vi "Test_Split.vi"() -> ()   [LabVIEW 2021]
panel:
  in  "OK Button":bool
  in  "milliseconds to wait":u32
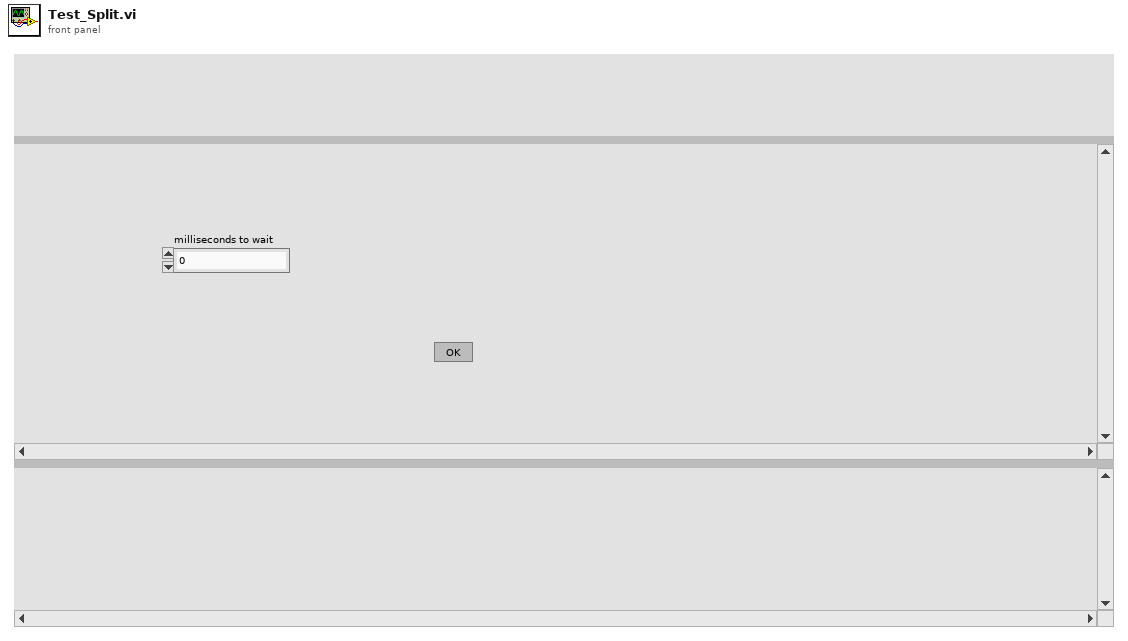
[diagram p1: front panel]
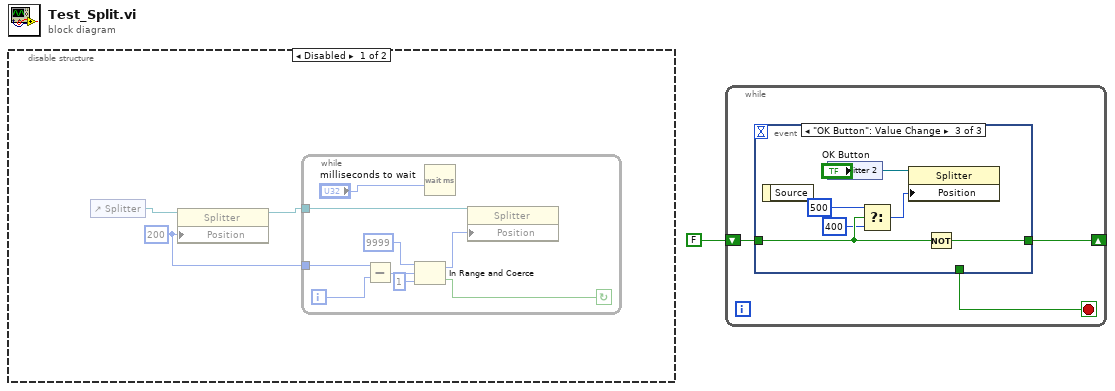
[diagram p0: block diagram]
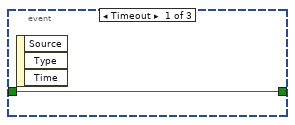
[diagram p2: hidden frame]
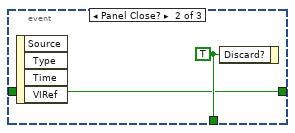
[diagram p3: hidden frame]
diagram:
  n1 = disable-structure shown="Disabled" {
    frame Disabled {
      w2 = 200 ("Splitter Position")
      n2 = control-ref of="Splitter"() -> (w4:refnum<vi>)
      n3 = property class="Splitter"(reference=w4, "Position"=w2) -> (reference out=w3:refnum<vi>)  [unwired: 1 in, 1 out]
      n4 = while {
        tunnel: w3 -> [w13]
        tunnel: w2 -> [w12]
        i -> [w11]
        stop <- w6 continue-if-true
        n5 = Subtract(x=w12, y=w11) -> (x-y=w10:i32)
        n6 = In Range and Coerce(upper limit=9999, x=w10, lower limit=1) -> (coerced(x)=w9:i32, In Range?=w6:bool)
        n7 = Wait (ms)(milliseconds to wait="milliseconds to wait") -> ()  [unwired: 1 out]
        n8 = property class="Splitter"(reference=w13, "Position"=w9) -> ()  [unwired: 1 in, 2 out]
      }
    }
    frame Enabled {
    }
  }
  n9 = while {
    shift-right: [w14] -> _
    shift-left: FALSE -> [w15]
    stop <- w16 stop-if-true
    n10 = event shown="[2] \"OK Button\": Value Change" {
      selector: _ -> [_ _ _]
      dyn-events: _ -> [_ _ _]
      timeout: _ -> [_ _ _]
      tunnel: [_ w19 _] -> w16
      tunnel: w15 -> [w17 w18 w24]
      tunnel: [w17 w18 w23] -> w14
      event Timeout {
        n11 = event-data() -> ()  [unwired: 1 in, 3 out]
      }
      event Panel Close? {
        w19 = TRUE ("Discard?")
        n12 = event-data() -> ()  [unwired: 1 in, 4 out]
        n13 = event-data("Discard?"=w19) -> ()  [unwired: 1 in, 1 out]
      }
      event "OK Button": Value Change {
        n14 = event-data() -> ()  [unwired: 1 in, 1 out]
        n15 = control-ref of="Splitter 2"() -> (w25:refnum<vi>)
        n16 = Select(t=500 ("Splitter Position"), s=w24, f=400) -> (s? t:f=w22:i32)
        n17 = property class="Splitter"(reference=w25, "Position"=w22) -> ()  [unwired: 1 in, 2 out]
        n18 = Not(x=w24) -> (.not. x?=w23:bool)
      }
    }
  }
